vi "Tree_Update Tree.vi"(4 "Close Items":bool, 6 "Disabled?":bool[](array[boolean]), 8 "error in":errorcluster, 9 "New Items":T1(array[cluster]), 10 "Show Changed":bool, 11 "TreeControl in":refnum<vi>) -> (0 "error out":errorcluster, 3 "TreeControl out":refnum<vi>)   [LabVIEW 2023]
doc: "Update tree with new items. If filtered, try to maintain position on change of show scripting/private."
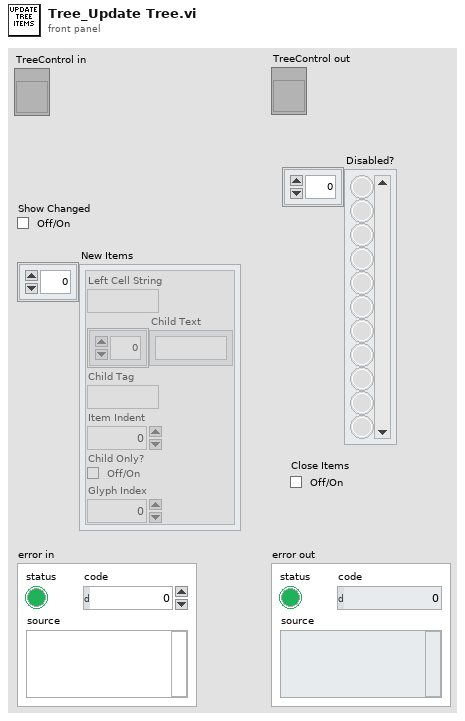
[diagram p1: front panel]
types:
  T1 = cluster{"Left Cell String":string, "Child Text":string[], "Child Tag":string, "Item Indent":i32, "Child Only?":bool, "Glyph Index":i32}[]
  T2 = typedef "LVNodeAndColumnTypeDef.ctl" = cluster{"Node":string, "Column":i32}
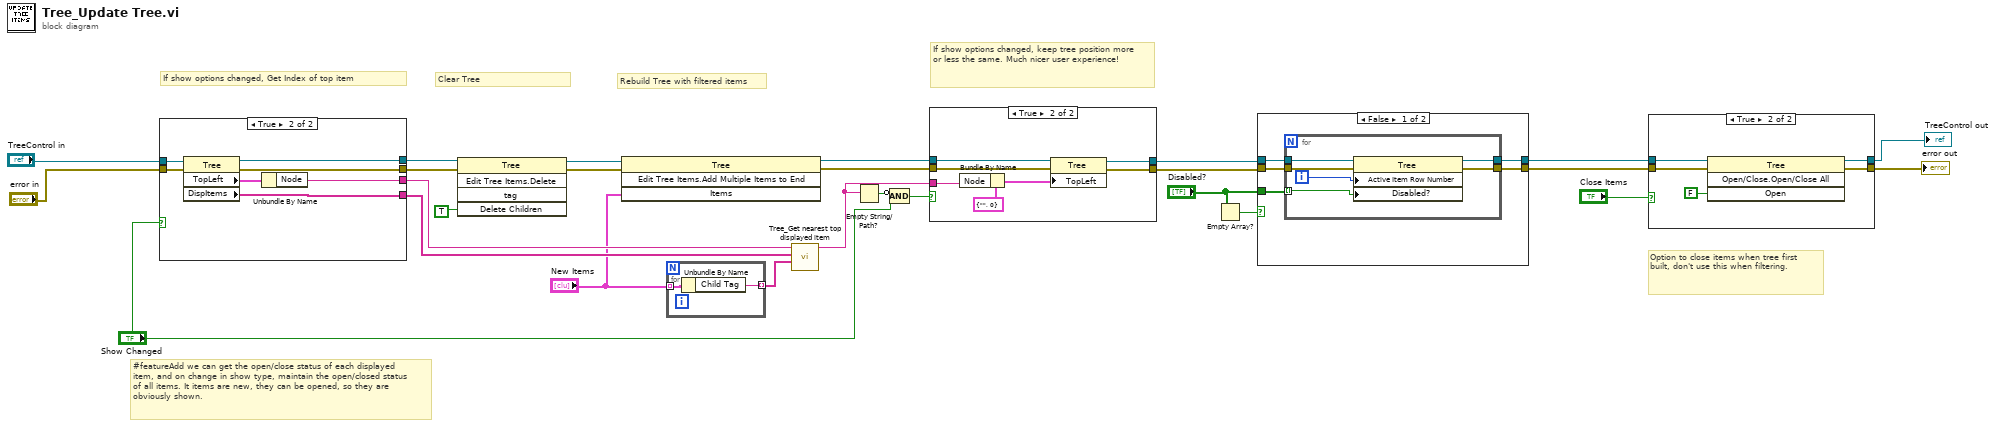
[diagram p0: block diagram]
diagram:
  # "#featureAdd we can get the open/close status of each displayed item, and on change in show type, maintain the open/closed status of all items. It items are new, they can be opened, so they are obviously shown."
  # "Option to close items when tree first built, don't use this when filtering."
  # "If show options changed, keep tree position more or less the same. Much nicer user experience!"
  # "Rebuild Tree with filtered items"
  # "Clear Tree"
  # "If show options changed, Get Index of top item"
  n1 = case shown="True" "Show Changed" {
    tunnel: "TreeControl in" -> [w27 w35]
    tunnel: "error in" -> [w28 w34]
    tunnel: [w27 w33] -> w17
    tunnel: [w28 w32] -> w18
    tunnel: [_ w30] -> w22
    tunnel: [_ w29] -> w21
    frame False {
    }
    frame True {
      n2 = property class="Tree"(reference=w35, error in=w34) -> (reference out=w33:refnum<vi>, error out=w32:errorcluster, "TopLeft"=w31:T2, "DispItems"=w29:string[])
      n3 = Unbundle By Name(w31) -> ("Node"=w30:string)
    }
  }
  n4 = invoke class="Tree" method="Edit Tree Items.Delete"(reference=w17, error in=w18, "Delete Children"=TRUE ("Delete Children?")) -> (reference out=w13:refnum<vi>, error out=w14:errorcluster)  [unwired: 2 in, 3 out]
  n5 = invoke class="Tree" method="Edit Tree Items.Add Multiple Items to End"(reference=w13, error in=w14, "Items"="New Items") -> (reference out=w19:refnum<vi>, error out=w20:errorcluster)  [unwired: 1 in, 2 out]
  n6 = for {
    tunnel: "New Items" -> [w37] mode=indexing
    tunnel: [w36] -> w10 mode=indexing
    n7 = Unbundle By Name(w37) -> ("Child Tag"=w36:string)
  }
  n8 = call "Tree_Get nearest top displayed item.vi"("Retained Tags"=w10, "Original Tags"=w21, "Top Tag In"=w22) -> ("Top Tag Out"=w23:string)  [unwired: 8 in]
  n9 = Empty String/Path?(string/path=w23) -> (empty?=w24:bool)
  n10 = Compound Arithmetic op=AND(invert w24, "Show Changed") -> (w25:bool)
  n11 = case shown="True" w25 {
    tunnel: w19 -> [w39 w46]
    tunnel: [w39 w45] -> w8
    tunnel: w20 -> [w38 w44]
    tunnel: [w38 w43] -> w7
    tunnel: w23 -> [_ w40]
    frame False {
    }
    frame True {
      n12 = Bundle By Name(cluster=cluster{"Node":string, "Column":i32} {"Node"="", "Column"=0} ("Top Left Visible Cell"), "Node"=w40) -> (w42:cluster{"Node":string, "Column":i32})
      n13 = property class="Tree"(reference=w46, error in=w44, "TopLeft"=w42) -> (reference out=w45:refnum<vi>, error out=w43:errorcluster)
    }
  }
  n14 = Empty Array?(array="Disabled?") -> (empty?=w9:bool)
  n15 = case shown="False" w9 {
    tunnel: w8 -> [w51 w59]
    tunnel: [w50 w59] -> w5
    tunnel: w7 -> [w49 w58]
    tunnel: [w48 w58] -> w4
    tunnel: "Disabled?" -> [w47 _]
    frame False {
      n16 = for {
        tunnel: w51 -> [w57]
        tunnel: [w55] -> w50
        tunnel: w49 -> [w54]
        tunnel: [w53] -> w48
        tunnel: w47 -> [w52] mode=indexing
        i -> [w56]
        n17 = property class="Tree"(reference=w57, error in=w54, "Active Item Row Number"=w56, "Disabled?"=w52) -> (reference out=w55:refnum<vi>, error out=w53:errorcluster)
      }
    }
    frame True {
    }
  }
  n18 = case shown="True" "Close Items" {
    tunnel: w5 -> [w61 w66]
    tunnel: w4 -> [w60 w65]
    tunnel: [w61 w64] -> w3
    tunnel: [w60 w63] -> w2
    frame False {
    }
    frame True {
      n19 = invoke class="Tree" method="Open/Close.Open/Close All"(reference=w66, error in=w65, "Open"=FALSE ("Open?")) -> (reference out=w64:refnum<vi>, error out=w63:errorcluster)  [unwired: 1 in, 2 out]
    }
  }
  "error out" <- w2
  "TreeControl out" <- w3
